vi "KundtsTube.vi"() -> ()   [LabVIEW 2015]
uses:
  <vilib>/Utility/file.llb/Write Delimited Spreadsheet (DBL).vi
panel:
  in  "Number of Samples":dbl=100000.0
  in  "Sampling rate (Hz)":dbl=100000.0
  in  "Amplitude":dbl=1.0
  in  "?":enum32{"Sweep", "Single"}(tab)
  in  "?":bool
  in  "Dwell Time (s)":dbl=1.0
  out "Sweep Waveform":dynamicdata(graph)=[{"t0"=timestamp(3530047799.6855407 s since 1904-01-01), "dt"=9.999999999999972e-06, "Y"=array[100000 elements], "attributes"=variant("NI_ChannelName"=variant(string "Voltage"), "NI_UnitDescription"=variant(string "Volts"))}] caption="Sine"
  out "Gain vs. Frequency":cluster{dbl[], dbl[]}(graph)
  in  "Frequency":dbl=1000.0
  out "Single Waveform":dynamicdata(graph)=[{"t0"=timestamp(3530045477.333027 s since 1904-01-01), "dt"=9.999999999999972e-06, "Y"=array[100000 elements], "attributes"=variant("NI_ChannelName"=variant(string "Voltage"), "NI_UnitDescription"=variant(string "Volts"))}] caption="Sine"
  out "Output":cluster{"Frequency":dbl, "RMS":dbl, "Gain":dbl}={"Frequency"=1000.0, "RMS"=0.10201554491722307, "Gain"=-16.816456267898705} {"RMS" format="%0.2f"}
  in  "stop":bool
  in  "Sweep Parameters":T1={"Minimum"=100.0, "Maximum"=10000.0, "Number of Points"=500.0, "Spacing"=0} {"Spacing" items=["Linear", "Logarithmic"]}
  # "This will sweep from min to max, pausing by the dwell time after each incriment."
  # "This will generate a single signal \nwith specified frequency"
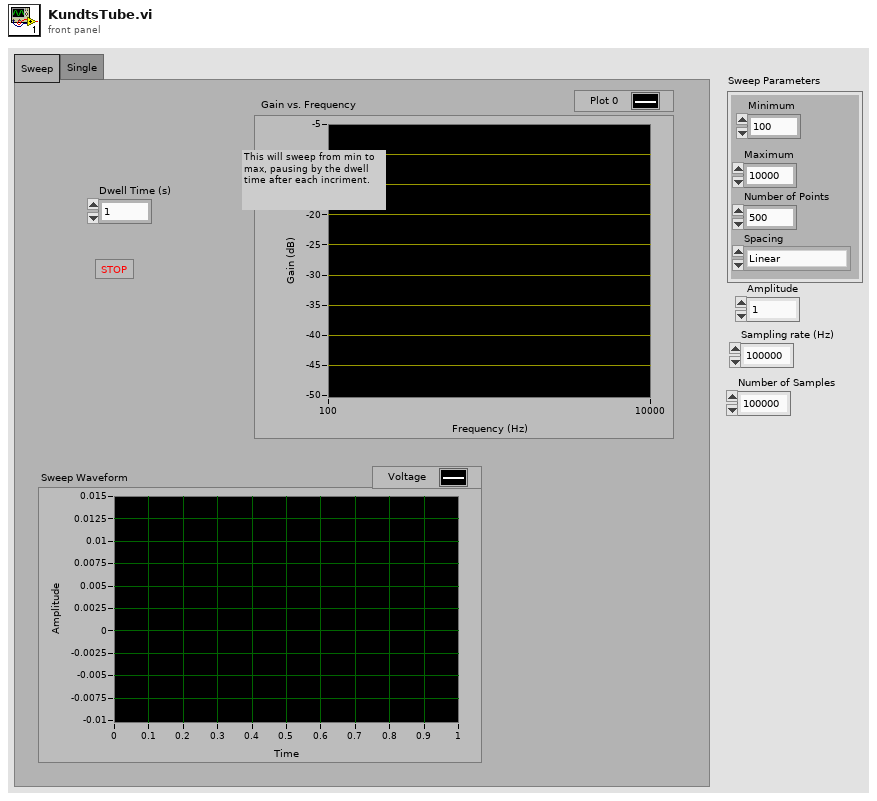
[diagram p1: front panel]
types:
  T1 = cluster{"Minimum":dbl, "Maximum":dbl, "Number of Points":dbl, "Spacing":u16}
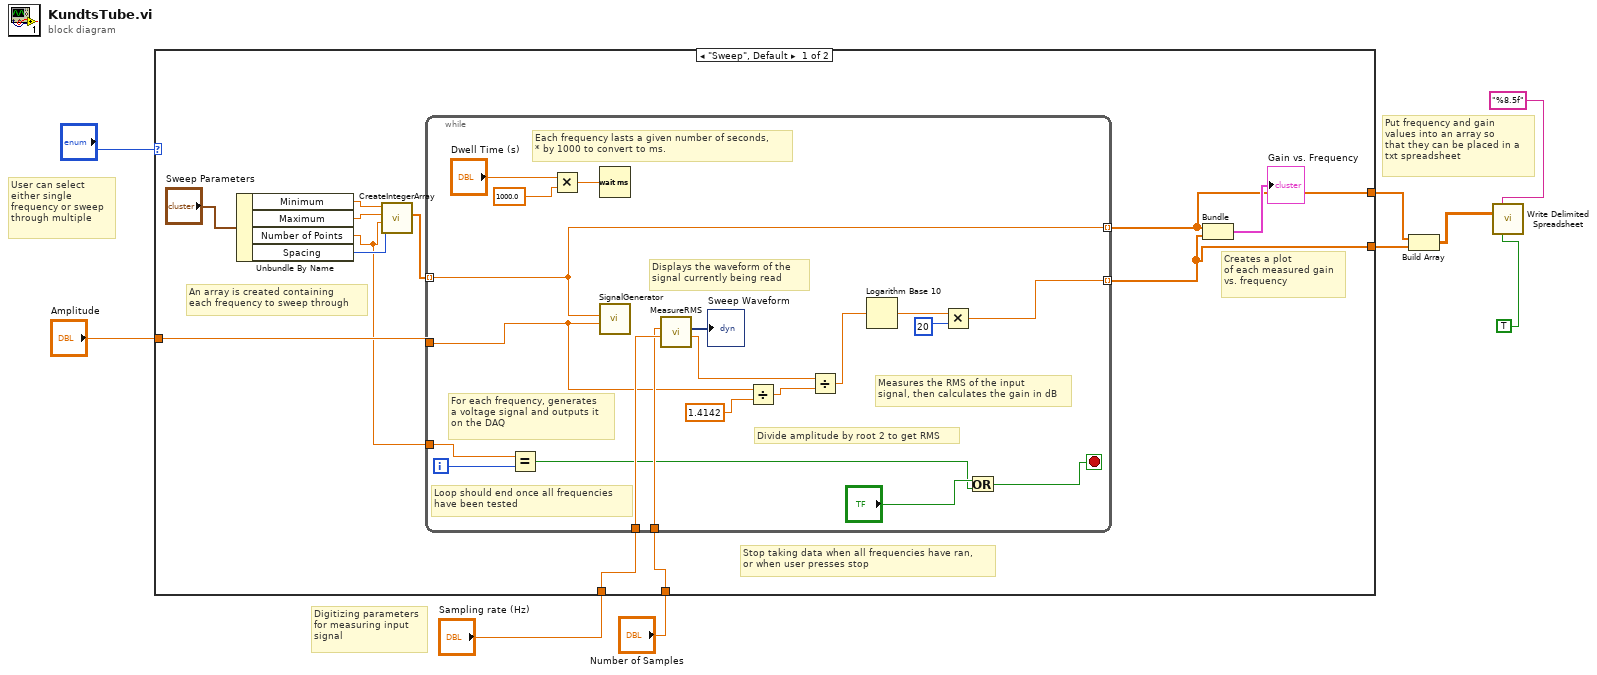
[diagram p0: block diagram]
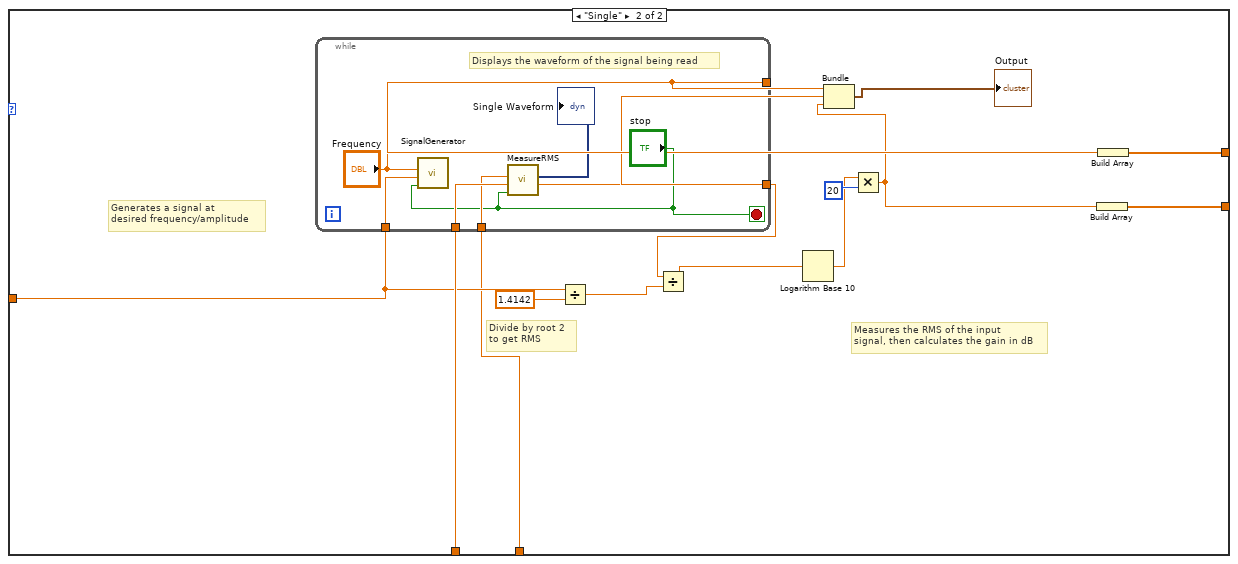
[diagram p2: hidden frame]
diagram:
  # "Put frequency and gain\nvalues into an array so \nthat they can be placed in a \ntxt spreadsheet"
  # "Digitizing parameters\nfor measuring input \nsignal"
  # "User can select\neither single \nfrequency or sweep\nthrough multiple"
  n1 = case shown="\"Sweep\", Default" "?" {
    tunnel: "Amplitude" -> [w20 w49]
    tunnel: "Sampling rate (Hz)" -> [w15 w55]
    tunnel: "Number of Samples" -> [w14 w48]
    tunnel: [w12 w45] -> w3
    tunnel: [w11 w43] -> w2
    frame "Sweep", Default {
      # "Stop taking data when all frequencies have ran, \nor when user presses stop"
      # "Creates a plot\nof each measured gain\nvs. frequency"
      # "An array is created containing\neach frequency to sweep through"
      n2 = Unbundle By Name("Sweep Parameters") -> ("Minimum"=w19:dbl, "Maximum"=w18:dbl, "Number of Points"=w10:dbl, "Spacing"=w17:u16)
      n3 = call "CreateIntegerArray.vi"("Spacing"=w17, "Number of Points"=w10, "Maximum"=w18, "Minimum"=w19) -> ("Output Array"=w16:dbl[])  [unwired: 7 in]
      n4 = while {
        tunnel: w20 -> [w31]
        tunnel: w16 -> [w32] mode=indexing
        tunnel: w15 -> [w39]
        tunnel: w14 -> [w38]
        tunnel: [w33] -> w11 mode=indexing
        tunnel: [w32] -> w12 mode=indexing
        tunnel: w10 -> [w25]
        i -> [w26]
        stop <- w23 stop-if-true
        # "Loop should end once all frequencies\nhave been tested"
        # "Divide amplitude by root 2 to get RMS"
        # "Displays the waveform of the \nsignal currently being read"
        # "Each frequency lasts a given number of seconds,\n* by 1000 to convert to ms."
        # "Measures the RMS of the input \nsignal, then calculates the gain in dB"
        # "For each frequency, generates\na voltage signal and outputs it \non the DAQ"
        n5 = Equal?(x=w25, y=w26) -> (x = y?=w22:bool)
        n6 = Multiply(x="Dwell Time (s)", y=1000.0) -> (x*y=w40:dbl)
        n7 = Wait (ms)(milliseconds to wait=w40) -> ()  [unwired: 1 out]
        n8 = call "SignalGenerator.vi"("Amplitude"=w31, "Frequency"=w32) -> ()  [unwired: 7 in, 2 out]
        n9 = call "MeasureRMS.vi"("Sampling rate (Hz)"=w39, "Number of Samples"=w38) -> ("RMS"=w37:dbl, "Waveform Graph"=→"Sweep Waveform":dynamicdata)  [unwired: 8 in]
        n10 = Divide(x=w31, y=1.4142) -> (x/y=w29:dbl)
        n11 = Divide(x=w37, y=w29) -> (x/y=w34:dbl)
        n12 = Logarithm Base 10(1:w34) -> (0:w35:dbl)
        n13 = Multiply(x=w35, y=20) -> (x*y=w33:dbl)
        n14 = Or(x="?", y=w22) -> (x .or. y?=w23:bool)
      }
      n15 = Bundle(w12, w11) -> (→"Gain vs. Frequency":cluster{dbl[], dbl[]})  [unwired: 1 in]
    }
    frame "Single" {
      # "Divide by root 2 \nto get RMS"
      # "Measures the RMS of the input \nsignal, then calculates the gain in dB"
      # "Generates a signal at \ndesired frequency/amplitude"
      n16 = while {
        tunnel: w55 -> [w61]
        tunnel: w49 -> [w60]
        tunnel: w48 -> [w59]
        tunnel: [w58] -> w42
        tunnel: ["Frequency"] -> w46
        stop <- "stop" stop-if-true
        # "Displays the waveform of the signal being read"
        n17 = call "SignalGenerator.vi"("stop"="stop", "Amplitude"=w60, "Frequency"="Frequency") -> ()  [unwired: 6 in, 2 out]
        n18 = call "MeasureRMS.vi"("stop"="stop", "Sampling rate (Hz)"=w61, "Number of Samples"=w59) -> ("RMS"=w58:dbl, "Waveform Graph"=→"Single Waveform":dynamicdata)  [unwired: 7 in]
      }
      n19 = Divide(x=w49, y=1.4142) -> (x/y=w50:dbl)
      n20 = Divide(x=w42, y=w50) -> (x/y=w52:dbl)
      n21 = Logarithm Base 10(1:w52) -> (0:w53:dbl)
      n22 = Multiply(x=w53, y=20) -> (x*y=w44:dbl)
      n23 = Bundle("Frequency"=w46, "RMS"=w42, w44) -> (→"Output":cluster{"Frequency":dbl, "RMS":dbl, dbl})  [unwired: 1 in]
      n24 = Build Array(w44) -> (w43:dbl[])
      n25 = Build Array(w46) -> (w45:dbl[])
    }
  }
  n26 = Build Array(w3, w2) -> (w1:dbl[][])
  n27 = call-poly <vilib>:"Write Delimited Spreadsheet.vi"("format (%.3f)"="%8.5f", "2D data"=w1, "transpose? (F)"=TRUE) -> ()  [unwired: 11 in, 2 out]
